vi "Collect-single-image.vi"(8 "error in (no error)":errorcluster, 11 "Config. params. ref. in":refnum<data-value>) -> (0 "error out":errorcluster, 1 "Image ok?":bool, 2 "Images array":u8[][][](array[numeric]), 3 "Config. params. ref.":refnum<data-value>)   [LabVIEW 2013, in "CameraVision.lvlib" / "CV-Configuration.lvclass"]
uses:
  CV-Configuration.lvclass
  CV-Configuration.lvclass/CV-Configuration.ctl
  Read Framegrabber DLL file.vi
  Read BoardHandle.vi
  Read DMA adresses.vi
  Read Image arrays.vi
  Read Camport array.vi
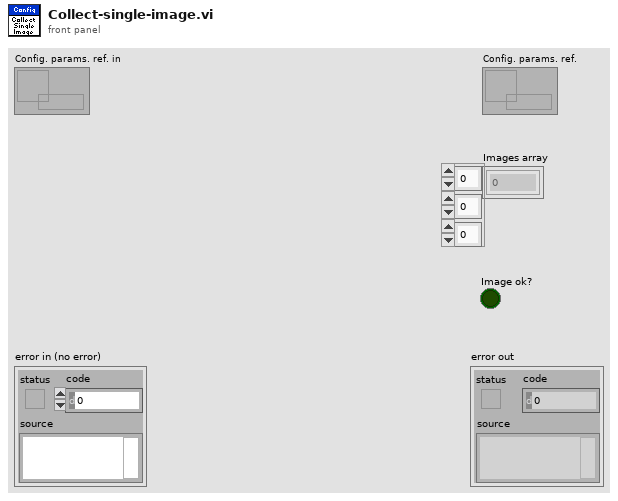
[diagram p1: front panel]
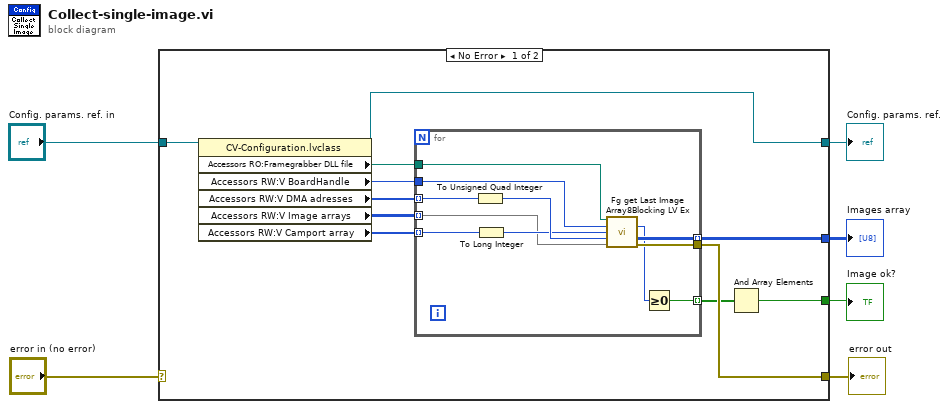
[diagram p0: block diagram]
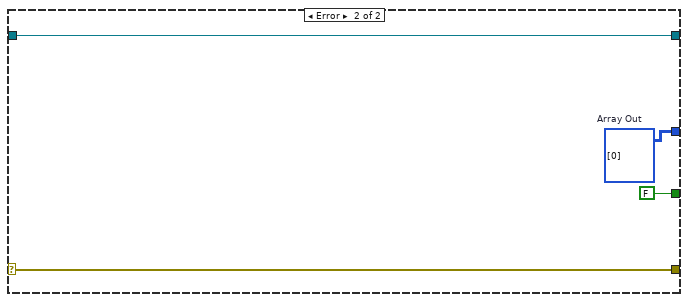
[diagram p2: hidden frame]
diagram:
  n1 = case shown="No Error" "error in (no error)" {
    selector: "error in (no error)" -> [_ w32]
    tunnel: [w9 w32] -> w5
    tunnel: "Config. params. ref. in" -> [w17 w31]
    tunnel: [w11 w31] -> w3
    tunnel: [w12 w30] -> w2
    tunnel: [w7 FALSE] -> w1
    frame No Error {
      n2 = property class="CV-Configuration.lvclass"(reference=w17) -> (reference out=w11:refnum<data-value>, "Accessors RO:Framegrabber DLL file"=w15:path, "Accessors RW:V BoardHandle"=w16:u64, "Accessors RW:V DMA adresses"=w14:i64[], "Accessors RW:V Image arrays"=w13:i8[][][], "Accessors RW:V Camport array"=w10:u32[])  [unwired: 1 in, 1 out]
      n3 = for {
        tunnel: w16 -> [w18]
        tunnel: w15 -> [w28]
        tunnel: w14 -> [w23] mode=indexing
        tunnel: w13 -> [w22] mode=indexing
        tunnel: [w26] -> w12 mode=indexing
        tunnel: w10 -> [w25] mode=indexing
        tunnel: [w21] -> w9
        tunnel: [w19] -> w8 mode=indexing
        n4 = To Unsigned Quad Integer(1:w23) -> (0:w27:u64)
        n5 = To Long Integer(number=w25) -> (32bit integer=w24:i32)
        n6 = call <userlib>:"Fg get Last Image Array8Blocking LV Ex.vi"("dll path in"=w28, "FgAddr"=w18, "CamPort"=w24, "DMAAddr"=w27, "Array"=w22) -> ("function return"=w20:u64, "Array Out"=w26:u8[][], "error out"=w21:errorcluster)  [unwired: 7 in, 1 out]
        n7 = Greater Or Equal To 0?(x=w20) -> (x >= 0?=w19:bool)
      }
      n8 = And Array Elements(Boolean array=w8) -> (logical AND=w7:bool)
    }
    frame Error {
      w30 = u8[][][] [[[0]]]  # Array Out
    }
  }
  "error out" <- w5
  "Config. params. ref." <- w3
  "Images array" <- w2
  "Image ok?" <- w1
